vi "XGT 연속읽기 (독립)01.vi"() -> ()   [LabVIEW 2012]
uses:
  <vilib>/Instr/_visa.llb/VISA Configure Serial Port (Instr).vi
panel:
  out "XY Graph":cluster{dbl[], dbl[]}(graph)
  out "배열 2":i32[][](array[numeric])
  in  "stop bits (10: 1 bit)":u16(ring)=10 caption="정지 비트(10: 1비트)" items=["1.0"=10, "1.5"=15, "2.0"=20]
  in  "parity (0:none)":enum16{"None", "Odd", "Even", "Mark", "Space"}(ring) caption="패리티(0:없음)"
  in  "data bits (8)":u16=8 caption="데이터 비트(8)" min=5 max=8 step=1
  in  "baud rate (9600)":u32=115200 caption="보 전송속도(9600)"
  in  "VISA resource name":refnum<visa-resource-name>="COM4" caption="VISA 리소스 이름"
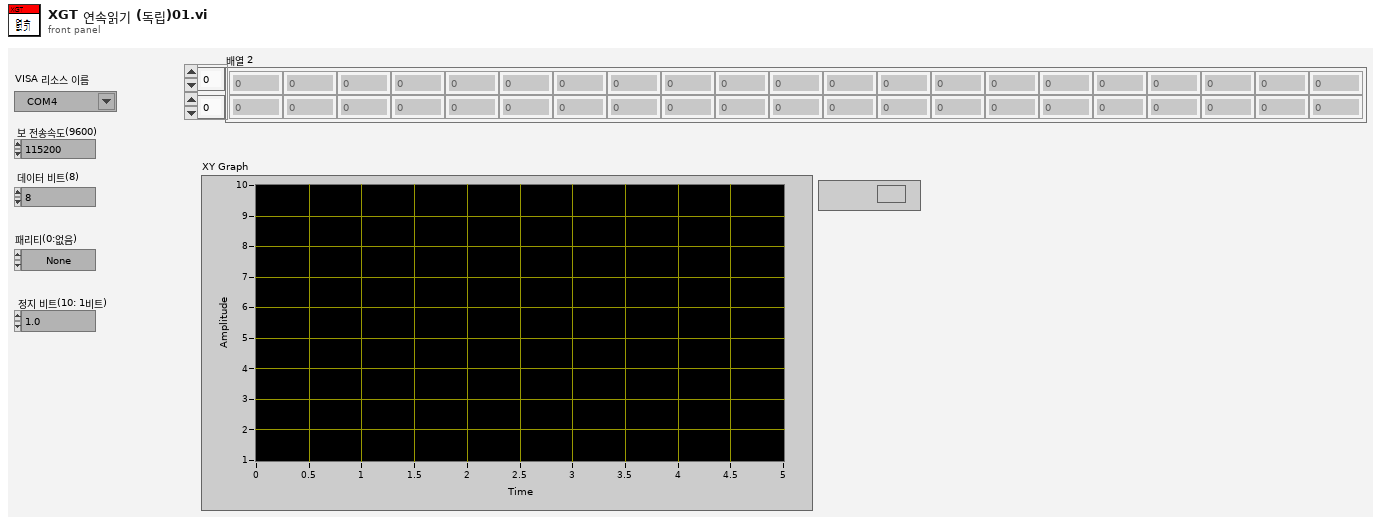
[diagram p1: front panel]
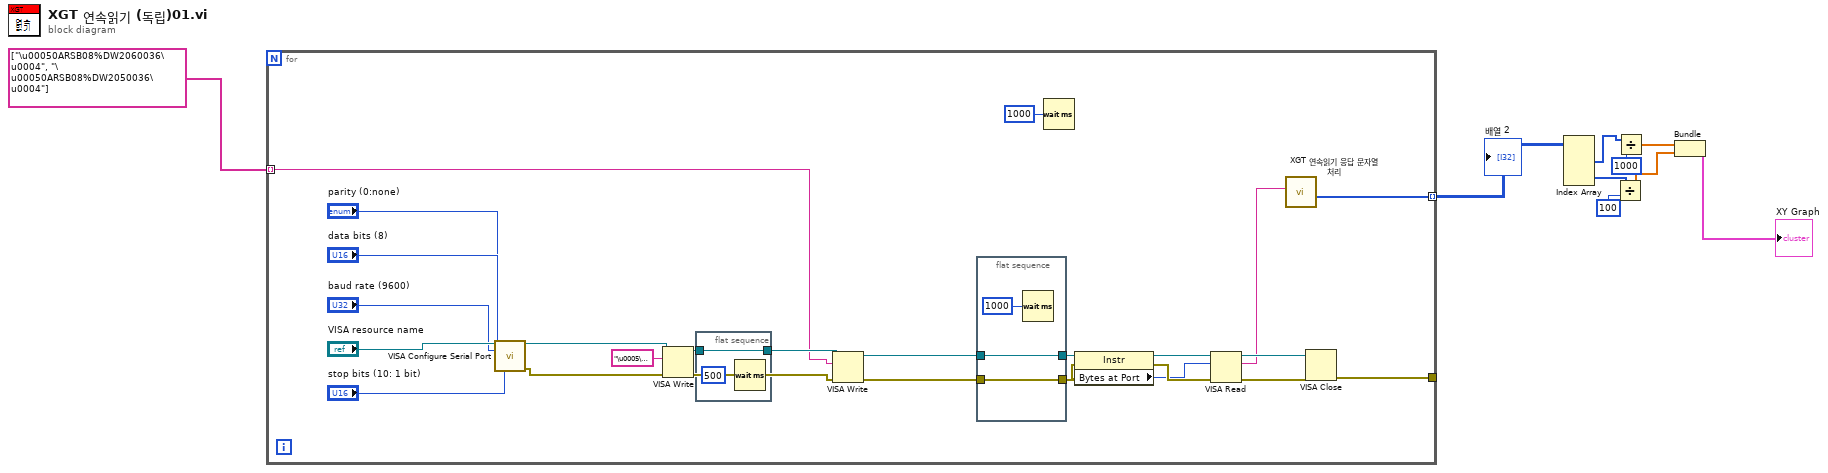
[diagram p0: block diagram]
diagram:
  n1 = for {
    tunnel: string[] ["\u00050ARSB08%DW2060036\u0004", "\u00050ARSB08%DW2050036\u0004"] -> [w13] mode=indexing
    tunnel: [w12] -> w9 mode=indexing
    tunnel: [w11] -> _
    n2 = call-poly "VISA Configure Serial Port"("VISA resource name"="VISA resource name", "baud rate (9600)"="baud rate (9600)", "data bits (8)"="data bits (8)", "parity (0:none)"="parity (0:none)", "stop bits (10: 1 bit)"="stop bits (10: 1 bit)") -> ("VISA resource name out"=w28:refnum<visa-resource-name>, "error out"=w27:errorcluster)  [unwired: 9 in]
    n3 = VISA Write(VISA resource name=w28, write buffer="\u0005\u0004", error in (no error)=w27) -> (VISA resource name out=w24:refnum<visa-resource-name>, error out=w25:errorcluster)  [unwired: 1 out]
    n4 = flat-sequence {
      tunnel: w24 -> [w39]
      tunnel: [w39] -> w23
      frame #0 {
        n5 = Wait (ms)(milliseconds to wait=u32 500) -> ()  [unwired: 1 out]
      }
    }
    n6 = VISA Write(VISA resource name=w23, write buffer=w13, error in (no error)=w25) -> (VISA resource name out=w20:refnum<visa-resource-name>, error out=w21:errorcluster)  [unwired: 1 out]
    n7 = flat-sequence {
      tunnel: w21 -> [w37]
      tunnel: [w37] -> w17
      tunnel: w20 -> [w36]
      tunnel: [w36] -> w18
      frame #0 {
        n8 = Wait (ms)(milliseconds to wait=u32 1000 ("대기 시간(ms)")) -> ()  [unwired: 1 out]
      }
    }
    n9 = Wait (ms)(milliseconds to wait=u32 1000) -> ()  [unwired: 1 out]
    n10 = property class="Instr"(reference=w18, error in=w17) -> (reference out=w16:refnum<visa-resource-name>, error out=w19:errorcluster, "Bytes at Port"=w15:u32)
    n11 = VISA Read(VISA resource name=w16, byte count=w15, error in (no error)=w19) -> (VISA resource name out=w26:refnum<visa-resource-name>, read buffer=w14:string, error out=w29:errorcluster)  [unwired: 1 out]
    n12 = call "XGT 연속읽기 응답 문자열 처리.vi"("응답"=w14) -> ("배열"=w12:i32[])  [unwired: 5 in, 5 out]
    n13 = VISA Close(VISA resource name=w26, error in (no error)=w29) -> (error out=w11:errorcluster)
  }
  "배열 2" <- w9
  n14 = Index Array(array=w9) -> (element #1=w6:i32[], element #2=w8:i32[])  [unwired: 4 in]
  n15 = Divide(x=w8, y=100) -> (x/y=w3:dbl[])
  n16 = Divide(x=w6, y=1000) -> (x/y=w4:dbl[])
  n17 = Bundle(w4, w3) -> (→"XY Graph":cluster{dbl[], dbl[]})  [unwired: 1 in]
